vi "FeedbackDecode_UpdateRegion.vi"(2 "EncodeClustIn":T1={"ParamsTable"=[], "Sel"=[], "Stim"=FALSE, "StimMode"=enum."Off", "StimStep"=[enum."1uA", enum."1uA", enum."Off"], "Jitter"=FALSE, "Pulse"=FALSE, "BFreq"=0.0, "BAmp"=0.0, "UEAArray"=[{"Boolean 1"=FALSE, "Boolean 2"=FALSE, "Boolean 3"=FALSE, "Boolean 4"=FALSE, "Boolean 5"=FALSE, "Boolean 6"=FALSE, "Boolean 7"=FALSE, "Boolean 8"=FALSE, "Boolean 9"=FALSE, "Boolean 10"=FALSE, "Boolean 11"=FALSE, "Boolean 12"=FALSE, "Boolean 13"=FALSE, "Boolean 14"=FALSE, "Boolean 15"=FALSE, "Boolean 16"=FALSE, "Boolean 17"=FALSE, "Boolean 18"=FALSE, "Boolean 19"=FALSE, "Boolean 20"=FALSE, "Boolean 21"=FALSE, "Boolean 22"=FALSE, "Boolean 23"=FALSE, "Boolean 24"=FALSE, "Boolean 25"=FALSE, "Boolean 26"=FALSE, "Boolean 27"=FALSE, "Boolean 28"=FALSE, "Boolean 29"=FALSE, "Boolean 30"=FALSE, "Boolean 31"=FALSE, "Boolean 32"=FALSE, "Boolean 33"=FALSE, "Boolean 34"=FALSE, "Boolean 35"=FALSE, "Boolean 36"=FALSE, "Boolean 37"=FALSE, "Boolean 38"=FALSE, "Boolean 39"=FALSE, "Boolean 40"=FALSE, "Boolean 41"=FALSE, "Boolean 42"=FALSE, "Boolean 43"=FALSE, "Boolean 44"=FALSE, "Boolean 45"=FALSE, "Boolean 46"=FALSE, "Boolean 47"=FALSE, "Boolean 48"=FALSE, "Boolean 49"=FALSE, "Boolean 50"=FALSE, "Boolean 51"=FALSE, "Boolean 52"=FALSE, "Boolean 53"=FALSE, "Boolean 54"=FALSE, "Boolean 55"=FALSE, "Boolean 56"=FALSE, "Boolean 57"=FALSE, "Boolean 58"=FALSE, "Boolean 59"=FALSE, "Boolean 60"=FALSE, "Boolean 61"=FALSE, "Boolean 62"=FALSE, "Boolean 63"=FALSE, "Boolean 64"=FALSE, "Boolean 65"=FALSE, "Boolean 66"=FALSE, "Boolean 67"=FALSE, "Boolean 68"=FALSE, "Boolean 69"=FALSE, "Boolean 70"=FALSE, "Boolean 71"=FALSE, "Boolean 72"=FALSE, "Boolean 73"=FALSE, "Boolean 74"=FALSE, "Boolean 75"=FALSE, "Boolean 76"=FALSE, "Boolean 77"=FALSE, "Boolean 78"=FALSE, "Boolean 79"=FALSE, "Boolean 80"=FALSE, "Boolean 81"=FALSE, "Boolean 82"=FALSE, "Boolean 83"=FALSE, "Boolean 84"=FALSE, "Boolean 85"=FALSE, "Boolean 86"=FALSE, "Boolean 87"=FALSE, "Boolean 88"=FALSE, "Boolean 89"=FALSE, "Boolean 90"=FALSE, "Boolean 91"=FALSE, "Boolean 92"=FALSE, "Boolean 93"=FALSE, "Boolean 94"=FALSE, "Boolean 95"=FALSE, "Boolean 96"=FALSE, "Boolean 97"=FALSE, "Boolean 98"=FALSE, "Boolean 99"=FALSE, "Boolean 100"=FALSE}, {"Boolean 1"=FALSE, "Boolean 2"=FALSE, "Boolean 3"=FALSE, "Boolean 4"=FALSE, "Boolean 5"=FALSE, "Boolean 6"=FALSE, "Boolean 7"=FALSE, "Boolean 8"=FALSE, "Boolean 9"=FALSE, "Boolean 10"=FALSE, "Boolean 11"=FALSE, "Boolean 12"=FALSE, "Boolean 13"=FALSE, "Boolean 14"=FALSE, "Boolean 15"=FALSE, "Boolean 16"=FALSE, "Boolean 17"=FALSE, "Boolean 18"=FALSE, "Boolean 19"=FALSE, "Boolean 20"=FALSE, "Boolean 21"=FALSE, "Boolean 22"=FALSE, "Boolean 23"=FALSE, "Boolean 24"=FALSE, "Boolean 25"=FALSE, "Boolean 26"=FALSE, "Boolean 27"=FALSE, "Boolean 28"=FALSE, "Boolean 29"=FALSE, "Boolean 30"=FALSE, "Boolean 31"=FALSE, "Boolean 32"=FALSE, "Boolean 33"=FALSE, "Boolean 34"=FALSE, "Boolean 35"=FALSE, "Boolean 36"=FALSE, "Boolean 37"=FALSE, "Boolean 38"=FALSE, "Boolean 39"=FALSE, "Boolean 40"=FALSE, "Boolean 41"=FALSE, "Boolean 42"=FALSE, "Boolean 43"=FALSE, "Boolean 44"=FALSE, "Boolean 45"=FALSE, "Boolean 46"=FALSE, "Boolean 47"=FALSE, "Boolean 48"=FALSE, "Boolean 49"=FALSE, "Boolean 50"=FALSE, "Boolean 51"=FALSE, "Boolean 52"=FALSE, "Boolean 53"=FALSE, "Boolean 54"=FALSE, "Boolean 55"=FALSE, "Boolean 56"=FALSE, "Boolean 57"=FALSE, "Boolean 58"=FALSE, "Boolean 59"=FALSE, "Boolean 60"=FALSE, "Boolean 61"=FALSE, "Boolean 62"=FALSE, "Boolean 63"=FALSE, "Boolean 64"=FALSE, "Boolean 65"=FALSE, "Boolean 66"=FALSE, "Boolean 67"=FALSE, "Boolean 68"=FALSE, "Boolean 69"=FALSE, "Boolean 70"=FALSE, "Boolean 71"=FALSE, "Boolean 72"=FALSE, "Boolean 73"=FALSE, "Boolean 74"=FALSE, "Boolean 75"=FALSE, "Boolean 76"=FALSE, "Boolean 77"=FALSE, "Boolean 78"=FALSE, "Boolean 79"=FALSE, "Boolean 80"=FALSE, "Boolean 81"=FALSE, "Boolean 82"=FALSE, "Boolean 83"=FALSE, "Boolean 84"=FALSE, "Boolean 85"=FALSE, "Boolean 86"=FALSE, "Boolean 87"=FALSE, "Boolean 88"=FALSE, "Boolean 89"=FALSE, "Boolean 90"=FALSE, "Boolean 91"=FALSE, "Boolean 92"=FALSE, "Boolean 93"=FALSE, "Boolean 94"=FALSE, "Boolean 95"=FALSE, "Boolean 96"=FALSE, "Boolean 97"=FALSE, "Boolean 98"=FALSE, "Boolean 99"=FALSE, "Boolean 100"=FALSE}], "AdjClust"={"Add"=FALSE, "Sub"=FALSE, "Val"=[1.0, 100.0, 10.0, 500.0, 0.2], "B"=[FALSE, FALSE, FALSE, FALSE, FALSE], "Inc+"=["x+1", "x+1", "x+10", "x+10", "x+0.1"], "Set"=FALSE, "LoadTable"=FALSE, "SaveTable"=FALSE, "ClearTable"=FALSE, "DeleteSel"=FALSE, "Inc-"=["x-1", "x-1", "x-10", "x-10", "x-0.1"]}, "PresetTable"=[], "SelPreset"=[], "SortClust"={"Region"=FALSE, "Receptor"=FALSE, "Electrode"=FALSE, "Min Amp"=FALSE, "Max Amp"=FALSE, "Min Freq"=FALSE, "Max Freq"=FALSE, "Duration"=FALSE}, "SelSort"={"Sel"=FALSE}, "PresetClust"={"Load"=FALSE, "Clear"=FALSE, "Save"=FALSE, "Del"=FALSE}, "RespClust"={"RespType"=enum."Sensor Map", "OpenResp"=FALSE}, "AmpLimit"=0.0, "FreqLimit"=0.0, "DurLimit"=0.0, "Wait Period"=0.0, "Train Period"=0.0} {"Train Period" min=0.0 max=100.0 step=0.1; "Wait Period" min=0.0 max=100.0 step=0.1; "DurLimit" min=0.0 max=1.0 step=0.01; "FreqLimit" min=0.0 max=500.0 step=1.0; "AmpLimit" min=0.0 max=100.0 step=1.0; "BAmp" min=0.0 max=100.0 step=1.0; "BFreq" min=0.0 max=100.0 step=1.0}, 3 "RegionStr":string) -> (0 "EncodeClustOut":T1={"ParamsTable"=[], "Sel"=[], "Stim"=FALSE, "StimMode"=enum."Off", "StimStep"=[enum."1uA", enum."1uA", enum."Off"], "Jitter"=FALSE, "Pulse"=FALSE, "BFreq"=0.0, "BAmp"=0.0, "UEAArray"=[{"Boolean 1"=FALSE, "Boolean 2"=FALSE, "Boolean 3"=FALSE, "Boolean 4"=FALSE, "Boolean 5"=FALSE, "Boolean 6"=FALSE, "Boolean 7"=FALSE, "Boolean 8"=FALSE, "Boolean 9"=FALSE, "Boolean 10"=FALSE, "Boolean 11"=FALSE, "Boolean 12"=FALSE, "Boolean 13"=FALSE, "Boolean 14"=FALSE, "Boolean 15"=FALSE, "Boolean 16"=FALSE, "Boolean 17"=FALSE, "Boolean 18"=FALSE, "Boolean 19"=FALSE, "Boolean 20"=FALSE, "Boolean 21"=FALSE, "Boolean 22"=FALSE, "Boolean 23"=FALSE, "Boolean 24"=FALSE, "Boolean 25"=FALSE, "Boolean 26"=FALSE, "Boolean 27"=FALSE, "Boolean 28"=FALSE, "Boolean 29"=FALSE, "Boolean 30"=FALSE, "Boolean 31"=FALSE, "Boolean 32"=FALSE, "Boolean 33"=FALSE, "Boolean 34"=FALSE, "Boolean 35"=FALSE, "Boolean 36"=FALSE, "Boolean 37"=FALSE, "Boolean 38"=FALSE, "Boolean 39"=FALSE, "Boolean 40"=FALSE, "Boolean 41"=FALSE, "Boolean 42"=FALSE, "Boolean 43"=FALSE, "Boolean 44"=FALSE, "Boolean 45"=FALSE, "Boolean 46"=FALSE, "Boolean 47"=FALSE, "Boolean 48"=FALSE, "Boolean 49"=FALSE, "Boolean 50"=FALSE, "Boolean 51"=FALSE, "Boolean 52"=FALSE, "Boolean 53"=FALSE, "Boolean 54"=FALSE, "Boolean 55"=FALSE, "Boolean 56"=FALSE, "Boolean 57"=FALSE, "Boolean 58"=FALSE, "Boolean 59"=FALSE, "Boolean 60"=FALSE, "Boolean 61"=FALSE, "Boolean 62"=FALSE, "Boolean 63"=FALSE, "Boolean 64"=FALSE, "Boolean 65"=FALSE, "Boolean 66"=FALSE, "Boolean 67"=FALSE, "Boolean 68"=FALSE, "Boolean 69"=FALSE, "Boolean 70"=FALSE, "Boolean 71"=FALSE, "Boolean 72"=FALSE, "Boolean 73"=FALSE, "Boolean 74"=FALSE, "Boolean 75"=FALSE, "Boolean 76"=FALSE, "Boolean 77"=FALSE, "Boolean 78"=FALSE, "Boolean 79"=FALSE, "Boolean 80"=FALSE, "Boolean 81"=FALSE, "Boolean 82"=FALSE, "Boolean 83"=FALSE, "Boolean 84"=FALSE, "Boolean 85"=FALSE, "Boolean 86"=FALSE, "Boolean 87"=FALSE, "Boolean 88"=FALSE, "Boolean 89"=FALSE, "Boolean 90"=FALSE, "Boolean 91"=FALSE, "Boolean 92"=FALSE, "Boolean 93"=FALSE, "Boolean 94"=FALSE, "Boolean 95"=FALSE, "Boolean 96"=FALSE, "Boolean 97"=FALSE, "Boolean 98"=FALSE, "Boolean 99"=FALSE, "Boolean 100"=FALSE}, {"Boolean 1"=FALSE, "Boolean 2"=FALSE, "Boolean 3"=FALSE, "Boolean 4"=FALSE, "Boolean 5"=FALSE, "Boolean 6"=FALSE, "Boolean 7"=FALSE, "Boolean 8"=FALSE, "Boolean 9"=FALSE, "Boolean 10"=FALSE, "Boolean 11"=FALSE, "Boolean 12"=FALSE, "Boolean 13"=FALSE, "Boolean 14"=FALSE, "Boolean 15"=FALSE, "Boolean 16"=FALSE, "Boolean 17"=FALSE, "Boolean 18"=FALSE, "Boolean 19"=FALSE, "Boolean 20"=FALSE, "Boolean 21"=FALSE, "Boolean 22"=FALSE, "Boolean 23"=FALSE, "Boolean 24"=FALSE, "Boolean 25"=FALSE, "Boolean 26"=FALSE, "Boolean 27"=FALSE, "Boolean 28"=FALSE, "Boolean 29"=FALSE, "Boolean 30"=FALSE, "Boolean 31"=FALSE, "Boolean 32"=FALSE, "Boolean 33"=FALSE, "Boolean 34"=FALSE, "Boolean 35"=FALSE, "Boolean 36"=FALSE, "Boolean 37"=FALSE, "Boolean 38"=FALSE, "Boolean 39"=FALSE, "Boolean 40"=FALSE, "Boolean 41"=FALSE, "Boolean 42"=FALSE, "Boolean 43"=FALSE, "Boolean 44"=FALSE, "Boolean 45"=FALSE, "Boolean 46"=FALSE, "Boolean 47"=FALSE, "Boolean 48"=FALSE, "Boolean 49"=FALSE, "Boolean 50"=FALSE, "Boolean 51"=FALSE, "Boolean 52"=FALSE, "Boolean 53"=FALSE, "Boolean 54"=FALSE, "Boolean 55"=FALSE, "Boolean 56"=FALSE, "Boolean 57"=FALSE, "Boolean 58"=FALSE, "Boolean 59"=FALSE, "Boolean 60"=FALSE, "Boolean 61"=FALSE, "Boolean 62"=FALSE, "Boolean 63"=FALSE, "Boolean 64"=FALSE, "Boolean 65"=FALSE, "Boolean 66"=FALSE, "Boolean 67"=FALSE, "Boolean 68"=FALSE, "Boolean 69"=FALSE, "Boolean 70"=FALSE, "Boolean 71"=FALSE, "Boolean 72"=FALSE, "Boolean 73"=FALSE, "Boolean 74"=FALSE, "Boolean 75"=FALSE, "Boolean 76"=FALSE, "Boolean 77"=FALSE, "Boolean 78"=FALSE, "Boolean 79"=FALSE, "Boolean 80"=FALSE, "Boolean 81"=FALSE, "Boolean 82"=FALSE, "Boolean 83"=FALSE, "Boolean 84"=FALSE, "Boolean 85"=FALSE, "Boolean 86"=FALSE, "Boolean 87"=FALSE, "Boolean 88"=FALSE, "Boolean 89"=FALSE, "Boolean 90"=FALSE, "Boolean 91"=FALSE, "Boolean 92"=FALSE, "Boolean 93"=FALSE, "Boolean 94"=FALSE, "Boolean 95"=FALSE, "Boolean 96"=FALSE, "Boolean 97"=FALSE, "Boolean 98"=FALSE, "Boolean 99"=FALSE, "Boolean 100"=FALSE}], "AdjClust"={"Add"=FALSE, "Sub"=FALSE, "Val"=[1.0, 100.0, 10.0, 500.0, 0.2], "B"=[FALSE, FALSE, FALSE, FALSE, FALSE], "Inc+"=["x+1", "x+1", "x+10", "x+10", "x+0.1"], "Set"=FALSE, "LoadTable"=FALSE, "SaveTable"=FALSE, "ClearTable"=FALSE, "DeleteSel"=FALSE, "Inc-"=["x-1", "x-1", "x-10", "x-10", "x-0.1"]}, "PresetTable"=[], "SelPreset"=[], "SortClust"={"Region"=FALSE, "Receptor"=FALSE, "Electrode"=FALSE, "Min Amp"=FALSE, "Max Amp"=FALSE, "Min Freq"=FALSE, "Max Freq"=FALSE, "Duration"=FALSE}, "SelSort"={"Sel"=FALSE}, "PresetClust"={"Load"=FALSE, "Clear"=FALSE, "Save"=FALSE, "Del"=FALSE}, "RespClust"={"RespType"=enum."Sensor Map", "OpenResp"=FALSE}, "AmpLimit"=0.0, "FreqLimit"=0.0, "DurLimit"=0.0, "Wait Period"=0.0, "Train Period"=0.0} {"Train Period" min=0.0 max=100.0 step=0.1; "Wait Period" min=0.0 max=100.0 step=0.1; "DurLimit" min=0.0 max=1.0 step=0.01; "FreqLimit" min=0.0 max=500.0 step=1.0; "AmpLimit" min=0.0 max=100.0 step=1.0; "BAmp" min=0.0 max=100.0 step=1.0; "BFreq" min=0.0 max=100.0 step=1.0})   [LabVIEW 2020]
uses:
  FeedbackDecode_EncodeClust.ctl
panel:
  # "Value"
  # "Inc-"
  # "Inc+"
  # "Min Amp"
  # "Max Amp"
  # "Min Freq"
  # "Max Freq"
  # "Duration"
  # "Value"
  # "Inc-"
  # "Inc+"
  # "Min Amp"
  # "Max Amp"
  # "Min Freq"
  # "Max Freq"
  # "Duration"
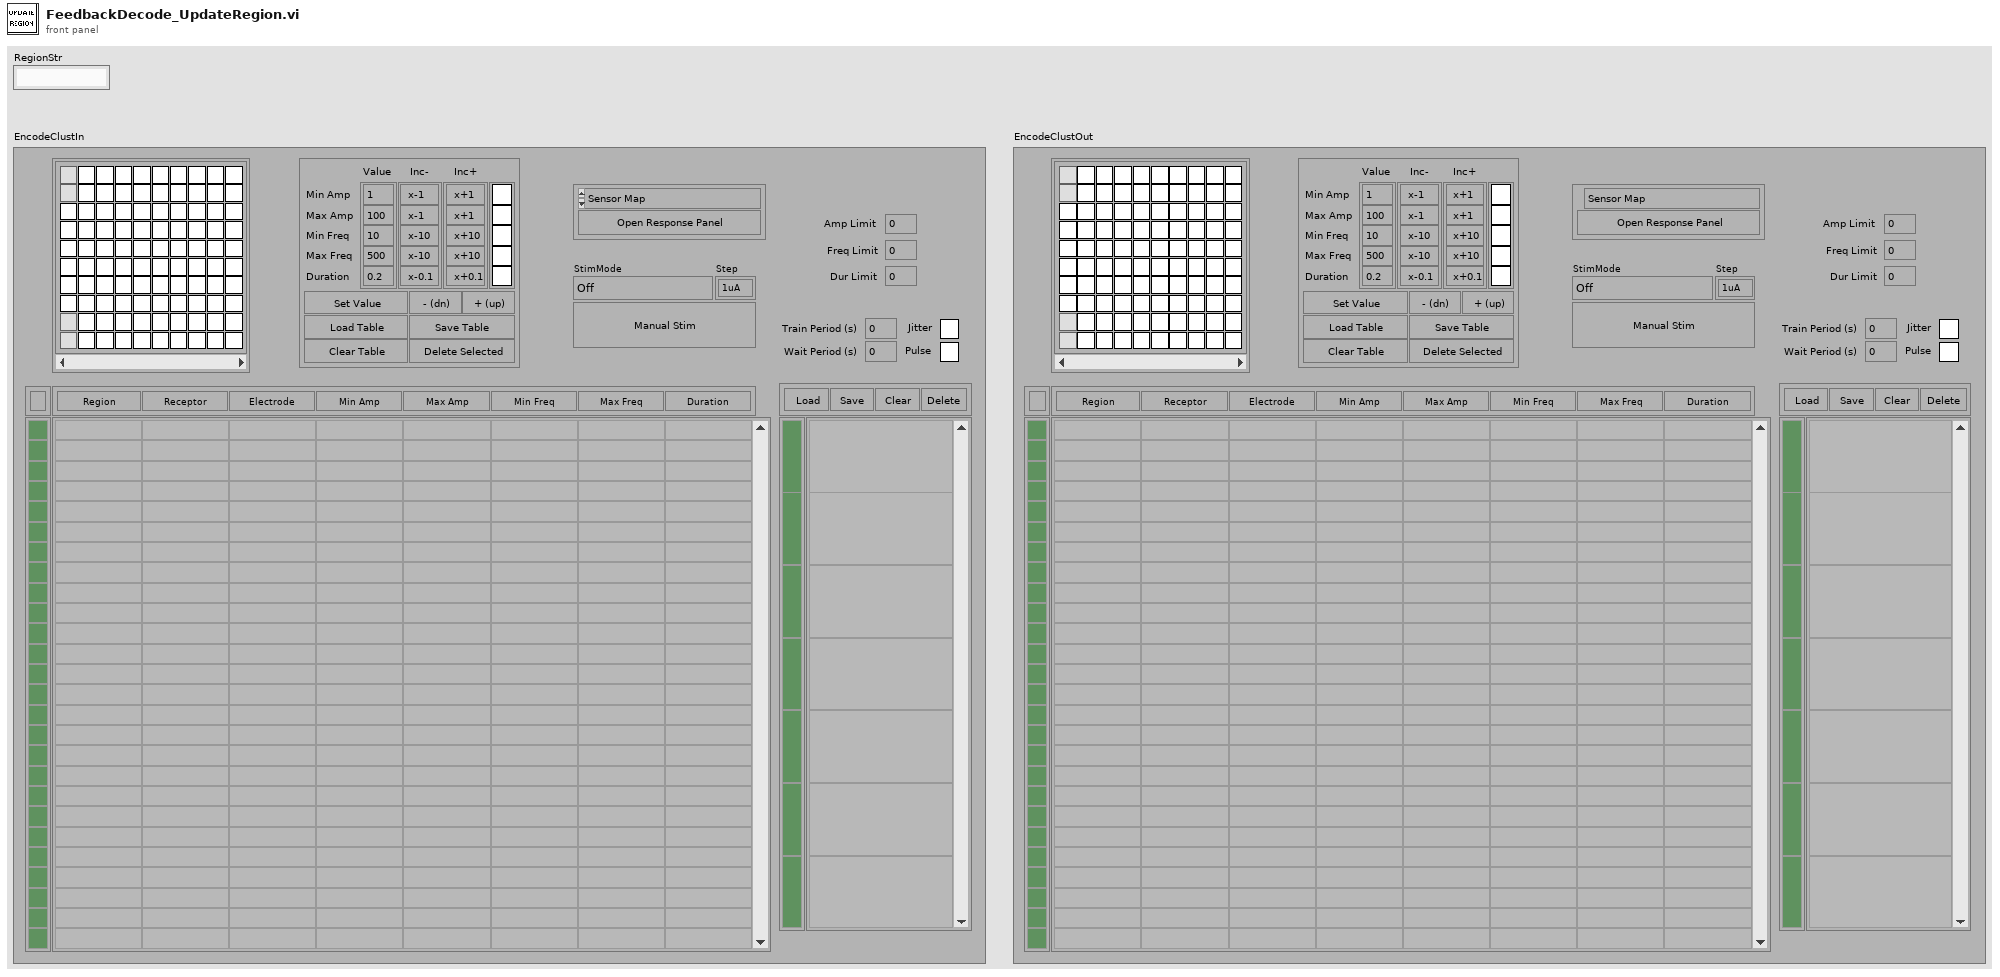
[diagram p1: front panel]
types:
  T1 = typedef "FeedbackDecode_EncodeClust.ctl" = cluster{"ParamsTable":string[][], "Sel":bool[], "Stim":bool, "StimMode":enum16{"Off", "Manual", "MSMS", "VRE", "3DHand", "DEKA", "Analog(DEKA)"}, "StimStep":enum16{"Off", "1uA", "2uA", "5uA", "10uA", "20uA", "30uA"}[], "Jitter":bool, "Pulse":bool, "BFreq":dbl, "BAmp":dbl, "UEAArray":cluster{"Boolean 1":bool, "Boolean 2":bool, "Boolean 3":bool, "Boolean 4":bool, "Boolean 5":bool, "Boolean 6":bool, "Boolean 7":bool, "Boolean 8":bool, "Boolean 9":bool, "Boolean 10":bool, "Boolean 11":bool, "Boolean 12":bool, "Boolean 13":bool, "Boolean 14":bool, "Boolean 15":bool, "Boolean 16":bool, "Boolean 17":bool, "Boolean 18":bool, "Boolean 19":bool, "Boolean 20":bool, "Boolean 21":bool, "Boolean 22":bool, "Boolean 23":bool, "Boolean 24":bool, "Boolean 25":bool, "Boolean 26":bool, "Boolean 27":bool, "Boolean 28":bool, "Boolean 29":bool, "Boolean 30":bool, "Boolean 31":bool, "Boolean 32":bool, "Boolean 33":bool, "Boolean 34":bool, "Boolean 35":bool, "Boolean 36":bool, "Boolean 37":bool, "Boolean 38":bool, "Boolean 39":bool, "Boolean 40":bool, "Boolean 41":bool, "Boolean 42":bool, "Boolean 43":bool, "Boolean 44":bool, "Boolean 45":bool, "Boolean 46":bool, "Boolean 47":bool, "Boolean 48":bool, "Boolean 49":bool, "Boolean 50":bool, "Boolean 51":bool, "Boolean 52":bool, "Boolean 53":bool, "Boolean 54":bool, "Boolean 55":bool, "Boolean 56":bool, "Boolean 57":bool, "Boolean 58":bool, "Boolean 59":bool, "Boolean 60":bool, "Boolean 61":bool, "Boolean 62":bool, "Boolean 63":bool, "Boolean 64":bool, "Boolean 65":bool, "Boolean 66":bool, "Boolean 67":bool, "Boolean 68":bool, "Boolean 69":bool, "Boolean 70":bool, "Boolean 71":bool, "Boolean 72":bool, "Boolean 73":bool, "Boolean 74":bool, "Boolean 75":bool, "Boolean 76":bool, "Boolean 77":bool, "Boolean 78":bool, "Boolean 79":bool, "Boolean 80":bool, "Boolean 81":bool, "Boolean 82":bool, "Boolean 83":bool, "Boolean 84":bool, "Boolean 85":bool, "Boolean 86":bool, "Boolean 87":bool, "Boolean 88":bool, "Boolean 89":bool, "Boolean 90":bool, "Boolean 91":bool, "Boolean 92":bool, "Boolean 93":bool, "Boolean 94":bool, "Boolean 95":bool, "Boolean 96":bool, "Boolean 97":bool, "Boolean 98":bool, "Boolean 99":bool, "Boolean 100":bool}[], "AdjClust":cluster{"Add":bool, "Sub":bool, "Val":dbl[], "B":bool[], "Inc+":string[], "Set":bool, "LoadTable":bool, "SaveTable":bool, "ClearTable":bool, "DeleteSel":bool, "Inc-":string[]}, "PresetTable":string[][], "SelPreset":bool[], "SortClust":cluster{"Region":bool, "Receptor":bool, "Electrode":bool, "Min Amp":bool, "Max Amp":bool, "Min Freq":bool, "Max Freq":bool, "Duration":bool}, "SelSort":cluster{"Sel":bool}, "PresetClust":cluster{"Load":bool, "Clear":bool, "Save":bool, "Del":bool}, "RespClust":cluster{"RespType":enum16{"Sensor Map", "Full Map"}, "OpenResp":bool}, "AmpLimit":dbl, "FreqLimit":dbl, "DurLimit":dbl, "Wait Period":dbl, "Train Period":dbl}
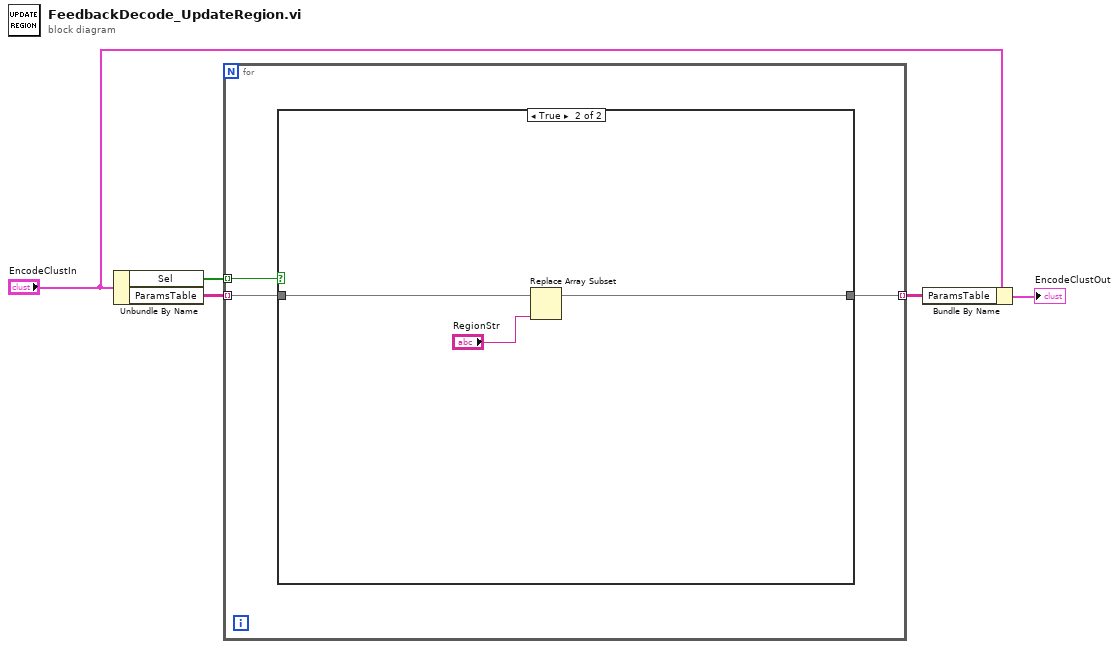
[diagram p0: block diagram]
diagram:
  n1 = Unbundle By Name("EncodeClustIn") -> ("Sel"=w5:bool[], "ParamsTable"=w4:string[][])
  n2 = for {
    tunnel: w5 -> [w8] mode=indexing
    tunnel: w4 -> [w7] mode=indexing
    tunnel: [w6] -> w2 mode=indexing
    n3 = case shown="True" w8 {
      tunnel: w7 -> [w9 w12]
      tunnel: [w9 w10] -> w6
      frame False {
      }
      frame True {
        n4 = Replace Array Subset(array=w12, new element="RegionStr") -> (w10:string[])  [unwired: 1 in]
      }
    }
  }
  n5 = Bundle By Name(cluster="EncodeClustIn", "ParamsTable"=w2) -> (→"EncodeClustOut":T1)
